vi "GetImageFromPackageCUID.vi"(10 "PackageCUID":string) -> (1 "Found":bool, 2 "path":path)   [LabVIEW 2016]
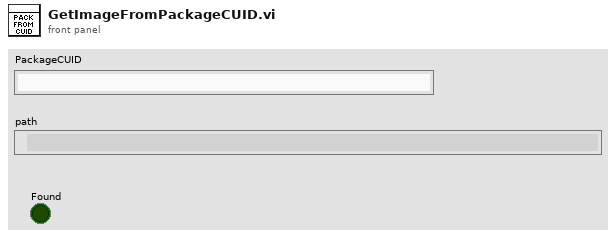
[diagram p1: front panel]
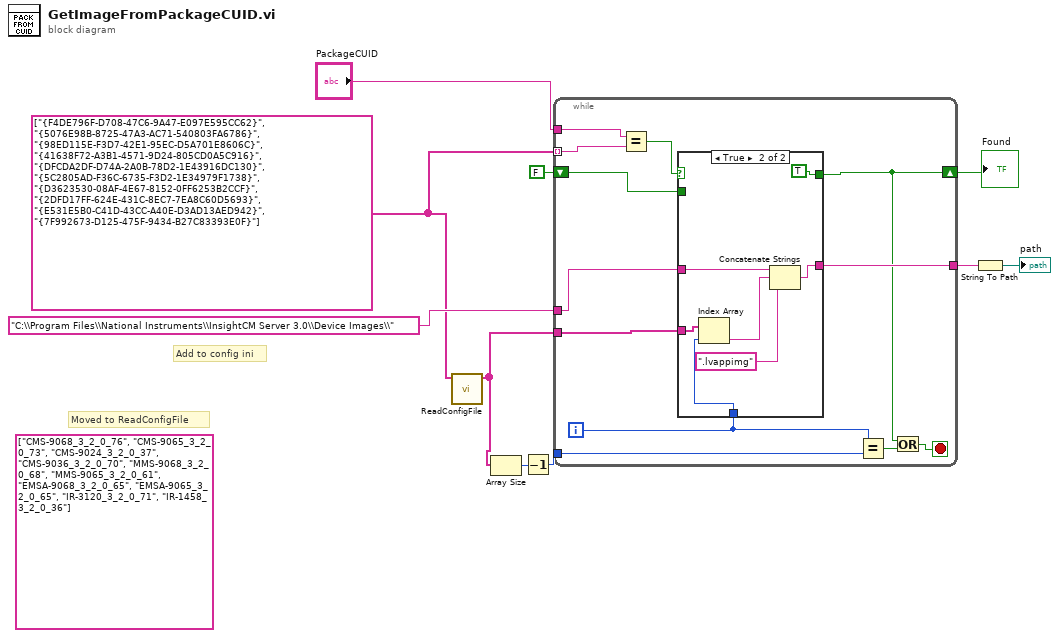
[diagram p0: block diagram]
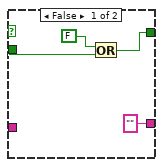
[diagram p2: hidden frame]
diagram:
  (unwired) string[] ["CMS-9068_3_2_0_76", "CMS-9065_3_2_0_73", "CMS-9024_3_2_0_37", "CMS-9036_3_2_0_70", "MMS-9068_3_2_0_68", "MMS-9065_3_2_0_61", "EMSA-9068_3_2_0_65", "EMSA-9065_3_2_0_65", "IR-3120_3_2_0_71", "IR-1458_3_2_0_36"] ("ImageVersion")
  w2 = string[] ["{F4DE796F-D708-47C6-9A47-E097E595CC62}", "{5076E98B-8725-47A3-AC71-540803FA6786}", "{98ED115E-F3D7-42E1-95EC-D5A701E8606C}", "{41638F72-A3B1-4571-9D24-805CD0A5C916}", "{DFCDA2DF-D74A-2A0B-78D2-1E43916DC130}", "{5C2805AD-F36C-6735-F3D2-1E34979F1738}", "{D3623530-08AF-4E67-8152-0FF6253B2CCF}", "{2DFD17FF-624E-431C-8EC7-7EA8C60D5693}", "{E531E5B0-C41D-43CC-A40E-D3AD13AED942}", "{7F992673-D125-475F-9434-B27C83393E0F}"] ("ImageName")
  # "Add to config ini"
  # "Moved to ReadConfigFile"
  n1 = call "ReadConfigFile.vi"("AppGUID"=w2) -> ("ImageName"=w1:string[])  [unwired: 10 in]
  n2 = Array Size(array=w1) -> (size(s)=w6:i32)
  n3 = Decrement(x=w6) -> (x-1=w5:i32)
  n4 = while {
    tunnel: w2 -> [w22] mode=indexing
    tunnel: "PackageCUID" -> [w21]
    tunnel: w1 -> [w17]
    shift-right: [w14] -> w8
    shift-left: FALSE -> [w19]
    tunnel: "C:\\Program Files\\National Instruments\\InsightCM Server 3.0\\Device Images\\" -> [w16]
    tunnel: [w18] -> w4
    tunnel: w5 -> [w11]
    i -> [w12]
    stop <- w15 stop-if-true
    n5 = Equal?(x=w21, y=w22) -> (x = y?=w20:bool)
    n6 = case shown="True" w20 {
      tunnel: w12 -> [_ w30]
      tunnel: [w26 TRUE] -> w14
      tunnel: w19 -> [w25 _]
      tunnel: ["" w27] -> w18
      tunnel: w17 -> [_ w31]
      tunnel: w16 -> [_ w28]
      frame False {
        n7 = Or(x=FALSE, y=w25) -> (x .or. y?=w26:bool)
      }
      frame True {
        n8 = Index Array(array=w31, index=w30) -> (element=w29:string)
        n9 = Concatenate Strings(w28, w29, ".lvappimg" ("string")) -> (w27:string)
      }
    }
    n10 = Equal?(x=w12, y=w11) -> (x = y?=w13:bool)
    n11 = Or(x=w14, y=w13) -> (x .or. y?=w15:bool)
  }
  "Found" <- w8
  n12 = String To Path(string=w4) -> (path=→"path":path)
